vi "Aspect Ratio Rectangle.vi"(11 "Bounds":dbl[](array[numeric])) -> (3 "Score":dbl)   [LabVIEW 2025]
doc: "This VI compares the calculated diameter and convex hull area to compare this shape to a half-hexagon."
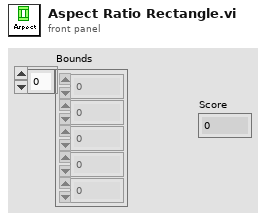
[diagram p1: front panel]
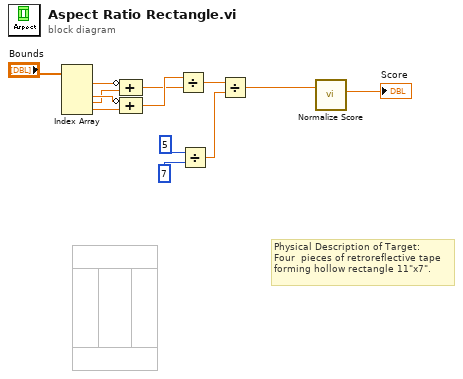
[diagram p0: block diagram]
diagram:
  # "Physical Description of Target:\nFour  pieces of retroreflective tape\nforming hollow rectangle 11\"x7\"."
  n1 = Index Array(array="Bounds") -> (element #1=w10:dbl, element #2=w9:dbl, element #3=w8:dbl, element #4=w11:dbl)  [unwired: 4 in]
  n2 = Compound Arithmetic op=ADD(invert w10, w8) -> (w6:dbl)
  n3 = Compound Arithmetic op=ADD(invert w9, w11) -> (w7:dbl)
  n4 = Divide(x=w7, y=w6) -> (x/y=w5:dbl)
  n5 = Divide(x=5, y=7) -> (x/y=w2:dbl)
  n6 = Divide(x=w5, y=w2) -> (x/y=w1:dbl)
  n7 = call "Normalize Score.vi"("Value"=w1) -> ("Score"=→"Score":dbl)  [unwired: 10 in]
